vi "InitializeBootstrap.vi"(8 "error in (no error)":errorcluster) -> (0 "error out":errorcluster, 2 "ProcessName":string, 3 "Qbus out":refnum<class "Qbus.lvclass">)   [LabVIEW 2017]
uses:
  <vilib>/addons/Qbus/Qbus.lvclass
  <vilib>/addons/InsightCM/Devices/Shared/Common/ServerComm/ServerComm.lvlib
  <vilib>/addons/TimerProcess/TimerProcess.lvlib
  <vilib>/addons/TraceLogger/TraceLogger.lvlib
  <vilib>/addons/InsightCM/Utilities/GlobalConfiguration/GlobalConfiguration.lvlib
  <vilib>/addons/SystemInfoProcess/SystemInfoProcess.lvlib
  <vilib>/addons/BlinkProcess/BlinkProcess.lvlib
  <vilib>/addons/InsightCM/Devices/Shared/Common/Controller/Controller.lvlib
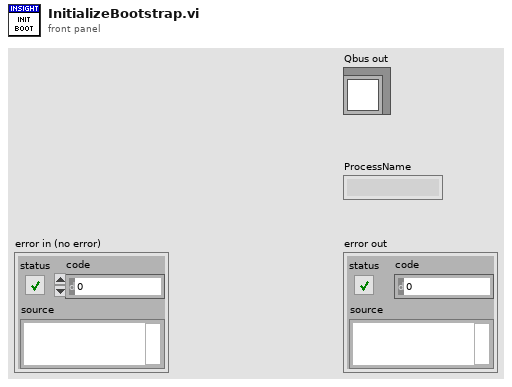
[diagram p1: front panel]
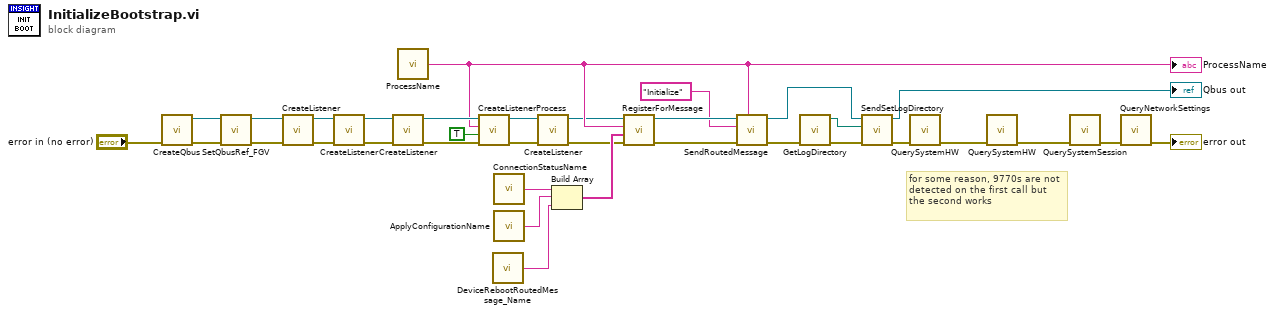
[diagram p0: block diagram]
diagram:
  # "for some reason, 9770s are not detected on the first call but the second works"
  n1 = call <vilib>:"CreateQbus.vi"("error in (no error)"="error in (no error)") -> ("error out"=w11:errorcluster, "Qbus"=w12:refnum<class "Qbus.lvclass">)  [unwired: 9 in]
  n2 = call <vilib>:"SetQbusRef_FGV.vi"("error in (no error)"=w11, "Qbus in"=w12) -> ("error out"=w9:errorcluster, "Qbus out"=w10:refnum<class "Qbus.lvclass">)  [unwired: 8 in]
  n3 = call <vilib>:"CreateListener.vi"("error in (no error)"=w9, "Qbus in"=w10) -> ("error out"=w34:errorcluster, "Qbus out"=w33:refnum<class "Qbus.lvclass">)  [unwired: 8 in]
  n4 = call <vilib>:"CreateListener.vi"("error in (no error)"=w34, "qbus in"=w33) -> ("error out"=w28:errorcluster, "qbus out"=w25:refnum<class "Qbus.lvclass">)  [unwired: 8 in]
  n5 = call <vilib>:"CreateListener.vi"("error in (no error)"=w28, "qbus in"=w25) -> ("error out"=w27:errorcluster, "qbus out"=w26:refnum<class "Qbus.lvclass">)  [unwired: 8 in]
  n6 = call <vilib>:"ProcessName.vi"() -> ("ProcessName"=w8:string)  [unwired: 5 in]
  "ProcessName" <- w8
  n7 = call <vilib>:"CreateListenerProcess.vi"("error in (no error)"=w27, "master"=TRUE ("Master"), "process name"=w8, "Qbus in"=w26) -> ("error in (no error)"=w4:errorcluster, "Qbus out"=w3:refnum<class "Qbus.lvclass">)  [unwired: 6 in]
  n8 = call <vilib>:"DeviceRebootRoutedMessage_Name.vi"() -> ("MessageName"=w7:string)  [unwired: 5 in]
  n9 = call <vilib>:"ConnectionStatusName.vi"() -> ("message name"=w32:string)  [unwired: 5 in]
  n10 = call <vilib>:"ApplyConfigurationName.vi"() -> ("message name"=w13:string)  [unwired: 5 in]
  n11 = call <vilib>:"CreateListener.vi"("error in (no error)"=w4, "Qbus in"=w3) -> ("error out"=w5:errorcluster, "Qbus out"=w6:refnum<class "Qbus.lvclass">)  [unwired: 8 in]
  n12 = Build Array(w32, w13, w7) -> (w31:string[])
  n13 = call <vilib>:"RegisterForMessage.vi"("error in (no error)"=w5, "message names"=w31, "process name"=w8, "Qbus in"=w6) -> ("error in (no error)"=w23:errorcluster, "Qbus out"=w24:refnum<class "Qbus.lvclass">)  [unwired: 6 in]
  n14 = call <vilib>:"SendRoutedMessage.vi"("listener process"=w8, "error in (no error)"=w23, "message name"="Initialize", "Qbus in"=w24) -> ("error in (no error)"=w19:errorcluster, "Qbus out"=w15:refnum<class "Qbus.lvclass">)  [unwired: 6 in]
  n15 = call <vilib>:"GetLogDirectory.vi"("error in (no error)"=w19) -> ("error out"=w20:errorcluster, "log dir"=w21:path)  [unwired: 9 in]
  n16 = call <vilib>:"SendSetLogDirectory.vi"("error in (no error)"=w20, "log directory"=w21, "qbus in"=w15) -> ("error out"=w18:errorcluster, "qbus out"=→"Qbus out":refnum<class "Qbus.lvclass">)  [unwired: 7 in]
  n17 = call <vilib>:"QuerySystemHW.vi"("error in (no error)"=w18) -> ("error out"=w2:errorcluster)  [unwired: 10 in]
  n18 = call <vilib>:"QuerySystemHW.vi"("error in (no error)"=w2) -> ("error out"=w1:errorcluster)  [unwired: 10 in]
  n19 = call <vilib>:"QuerySystemSession.vi"("error in (no error)"=w1) -> ("error out"=w17:errorcluster)  [unwired: 10 in]
  n20 = call <vilib>:"QueryNetworkSettings.vi"("error in (no error)"=w17) -> ("error out"=→"error out":errorcluster)  [unwired: 10 in]
